vi "Calc Type.vi"(11 "Calculation in":refnum<class "Calculation.lvclass">) -> (2 "Calc Type":string)   [LabVIEW 2020, in "VolatusCalcs.lvlib" / "Calculation.lvclass"]
uses:
  Calculation.lvclass
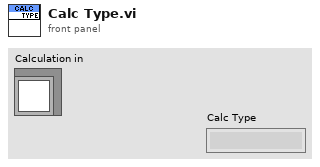
[diagram p1: front panel]
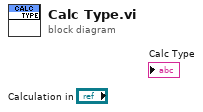
[diagram p0: block diagram]
diagram:
